vi "Write Return Deactivate Device Msg.vi"(10 "Return Deactivate Device Msg":refnum<class "Return Device Control Msg.lvclass">, 11 "Optimization in":refnum<class "Optimization.lvclass">) -> (3 "Optimization out":refnum<class "Optimization.lvclass">)   [LabVIEW 2016, in "Optimization Framework.lvlib" / "Optimization.lvclass"]
uses:
  Optimization.lvclass
  Optimization Messages/Return Device Control Msg/Return Device Control Msg.lvclass
  Optimization.lvclass/Optimization.ctl
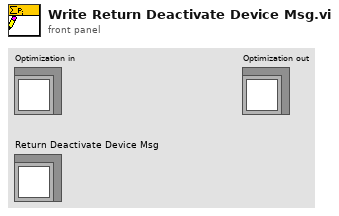
[diagram p1: front panel]
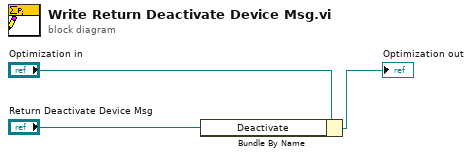
[diagram p0: block diagram]
diagram:
  n1 = Bundle By Name(cluster="Optimization in", "Deactivate"="Return Deactivate Device Msg") -> (→"Optimization out":refnum<class "Optimization.lvclass">)
